vi "PH_gentec_Powermeter.set Range.vi"(0 "i ref in":refnum<vi>, 2 "VISA resource in":refnum<visa-resource-name>, 4 "Device error in":errorcluster, 5 "error in":errorcluster) -> (13 "Settings changed?":bool, 14 "i ref out":refnum<vi>, 15 "Timeout":bool, 16 "VISA resource out":refnum<visa-resource-name>, 17 "Error Message":string, 18 "Device error out":errorcluster, 19 "error out":errorcluster)   [LabVIEW 2014, in "PH_gentec_Powermeter.lvlib"]
doc: "This VI sets the range of the powermeter. Then the value verified by the powermeter is passed to own attributes and the GUI element."
uses:
  PH_gentec_Powermeter.lvlib
  instr.lib/gentec-SOLO-PE/Driver/Type Defs/gentec-SOLO-PE.Zero Offset.ctl
  instr.lib/gentec-SOLO-PE/gentec-SOLO-PE - Driver.lvlib
  PH_Basics/PH_Powermeter_BaseClass/PH_Powermeter_BaseClass.lvlib
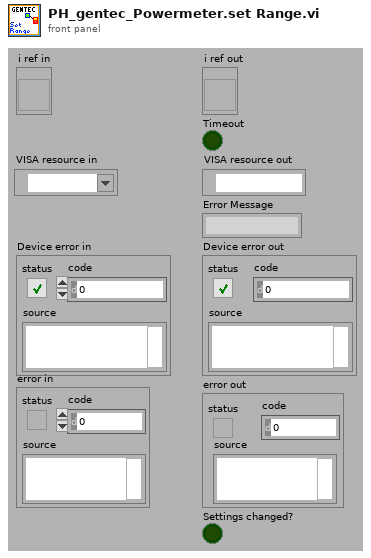
[diagram p1: front panel]
types:
  T1 = typedef "PH_Powermeter_BaseClass.lvlib/PH_Powermeter_BaseClass.i attribute.ctl" = cluster{"GUI References":T2, "Connection":T3, "Head Attributes":T5, "VISA resource":refnum<visa-resource-name>, "Energy":T6, "Service ID Energy":i32, "Wanted Settings":T7, "Current Settings":T7}
  T2 = typedef "PH_Powermeter_BaseClass.lvlib/PH_Powermeter_BaseClass.GUI Refs.ctl" = cluster{"Head Attributes":refnum<vi>, "Energy":refnum<vi>, "Connection":refnum<vi>, "VISA Resource":refnum<vi>, "Energy evolution":refnum<vi>, "Scaling Factor":refnum<vi>, "Range":refnum<vi>, "Wavelength":refnum<vi>, "Trigger Level":refnum<vi>, "Wanted Settings":refnum<vi>, "Current Settings":refnum<vi>}
  T3 = typedef "PH_Powermeter_BaseClass.lvlib/PH_Powermeter_BaseClass.Connection.ctl" = cluster{"failed checks":i8, "Timeout":bool, "Data read":string, "Failure":bool, "Error":bool, "State":T4}
  T4 = typedef "PH_Powermeter_BaseClass.lvlib/PH_Powermeter_BaseClass.State.ctl" = enum32{"off", "operating", "opened", "checked", "connected", "Sets to change", "running"}
  T5 = typedef "PH_Powermeter_BaseClass.lvlib/PH_Powermeter_BaseClass.Head Attributes.ctl" = cluster{"Instrument Type":string, "Head Version":string, "Head Name":string, "Serial Number":string, "Firmware":string, "Sensor Type":string, "MinimumRange":u32, "Maximum Range":u32, "Min Wavelength":i32, "Max Wavelength":i32}
  T6 = typedef "PH_Powermeter_BaseClass.lvlib/PH_Powermeter_BaseClass.Energy.ctl" = cluster{"current Value":dbl, "unscaled":dbl, "Scaling Factor":dbl}
  T7 = typedef "PH_Powermeter_BaseClass.lvlib/PH_gentec_BaseClass.Head Settings.ctl" = cluster{"Trigger Level":dbl, "Wavelength":u32, "Range":u32}
  T8 = typedef "gentec-SOLO-PE - Driver.lvlib/gentec-SOLO-PE.Zero Offset.ctl" = u32
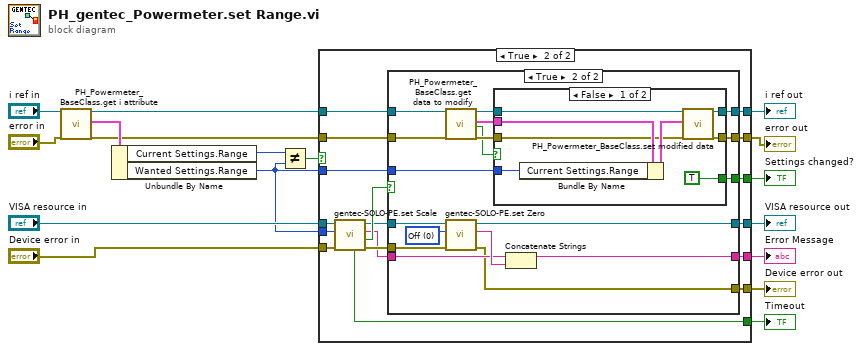
[diagram p0: block diagram]
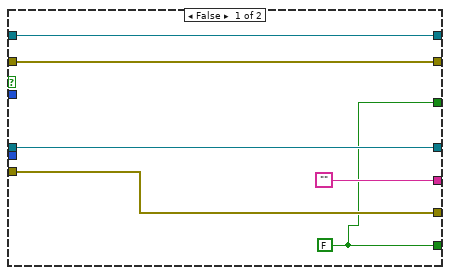
[diagram p2: hidden frame]
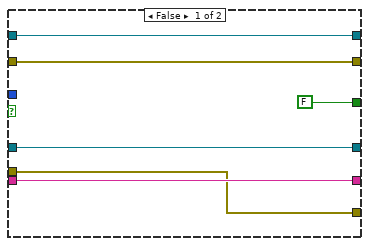
[diagram p3: hidden frame]
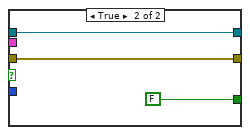
[diagram p4: hidden frame]
diagram:
  n1 = call "PH_Powermeter_BaseClass.get i attribute.vi"("i ref in"="i ref in", "error in (no error)"="error in") -> ("i ref out"=w10:refnum<vi>, "i attribute"=w13:T1, "error out"=w9:errorcluster)  [unwired: 15 in]
  n2 = Unbundle By Name(w13) -> ("Current Settings.Range"=w12:u32, "Wanted Settings.Range"=w4:u32)
  n3 = Not Equal?(x=w12, y=w4) -> (x != y?=w7:bool)
  n4 = case shown="True" w7 {
    tunnel: [w23 w40] -> w17
    tunnel: [w22 w39] -> w15
    tunnel: w4 -> [_ w35]
    tunnel: "VISA resource in" -> [w21 w36]
    tunnel: w10 -> [w23 w38]
    tunnel: w9 -> [w22 w34]
    tunnel: [w21 w25] -> w8
    tunnel: [w20 w24] -> w6
    tunnel: "Device error in" -> [w20 w37]
    tunnel: w4 -> [_ w33]
    tunnel: ["" w26] -> w2
    tunnel: [w18 w31] -> w3
    tunnel: [w18 w30] -> w1
    frame False {
      w18 = FALSE ("Timeout")
    }
    frame True {
      n5 = call "gentec-SOLO-PE.set Scale.vi"("error in (no error)"=w37, "Scale"=w35, "VISA Refnum in"=w36) -> ("error out"=w28:errorcluster, "Acknoledged?"=w32:bool, "Error"=w27:string, "VISA Refnum out"=w29:refnum<visa-resource-name>, "Timeout"=w31:bool)  [unwired: 4 in]
      n6 = case shown="True" w32 {
        tunnel: [w46 w60] -> w40
        tunnel: [w45 w59] -> w39
        tunnel: w38 -> [w46 w58]
        tunnel: w34 -> [w45 w57]
        tunnel: w33 -> [_ w56]
        tunnel: [FALSE w55] -> w30
        tunnel: w29 -> [w42 w54]
        tunnel: w28 -> [w41 w53]
        tunnel: w27 -> [w43 w51]
        tunnel: [w43 w50] -> w26
        tunnel: [w42 w49] -> w25
        tunnel: [w41 w48] -> w24
        frame False {
        }
        frame True {
          w47 = T8 0 items=["Off", "On", "Undo"] ("Zero Offset Operation")
          n7 = call "PH_Powermeter_BaseClass.get data to modify.vi"("i ref in"=w58, "error in (no error)"=w57) -> ("i ref out"=w64:refnum<vi>, "i attribute"=w63:T1, "timed out"=w61:bool, "error out"=w62:errorcluster)  [unwired: 14 in]
          n8 = call "gentec-SOLO-PE.set Zero.vi"("error in (no error)"=w53, "Zero Offset Operation"=w47, "VISA Refnum in"=w54) -> ("error out"=w48:errorcluster, "Error"=w52:string, "VISA Refnum out"=w49:refnum<visa-resource-name>)  [unwired: 4 in, 2 out]
          n9 = case shown="False" w61 {
            tunnel: w62 -> [w69 w74]
            tunnel: w64 -> [w72 w75]
            tunnel: [w66 w75] -> w60
            tunnel: [w65 w74] -> w59
            tunnel: w63 -> [w71 _]
            tunnel: w56 -> [w68 _]
            tunnel: [TRUE FALSE] -> w55
            frame False {
              n10 = Bundle By Name(cluster=w71, "Current Settings.Range"=w68) -> (w70:T1)
              n11 = call "PH_Powermeter_BaseClass.set modified data.vi"("i ref in"=w72, "i attribute"=w70, "error in (no error)"=w69) -> ("i ref out"=w66:refnum<vi>, "error out"=w65:errorcluster)  [unwired: 15 in]
            }
            frame True {
            }
          }
          n12 = Concatenate Strings(w51, w52) -> (w50:string)
        }
      }
    }
  }
  "error out" <- w15
  "i ref out" <- w17
  "VISA resource out" <- w8
  "Device error out" <- w6
  "Timeout" <- w3
  "Error Message" <- w2
  "Settings changed?" <- w1
